vi "UpdateZones.vi"(0 "object in":refnum<class "Team.lvclass">, 2 "Robots":refnum<class "Robot.lvclass">[](array[class]), 5 "error in (no error)":errorcluster) -> (14 "object out":refnum<class "Team.lvclass">, 19 "error out":errorcluster)   [LabVIEW 2023, in "Team.lvclass"]
uses:
  Team.lvclass
  Robot_class/Robot.lvclass
  Team.lvclass/Team.ctl
  Zone_class/Zone.lvclass
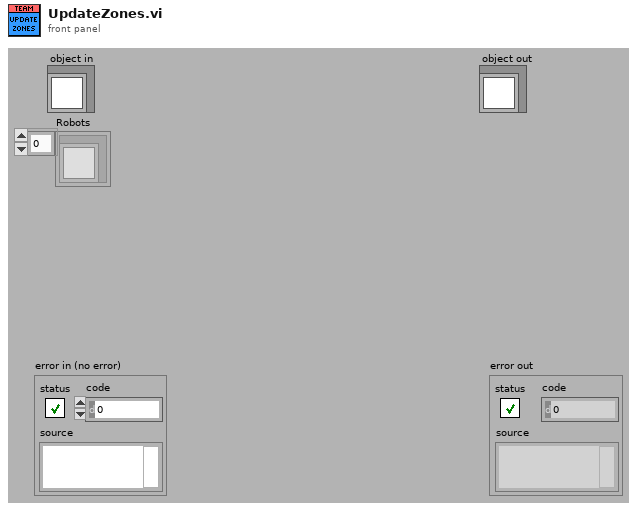
[diagram p1: front panel]
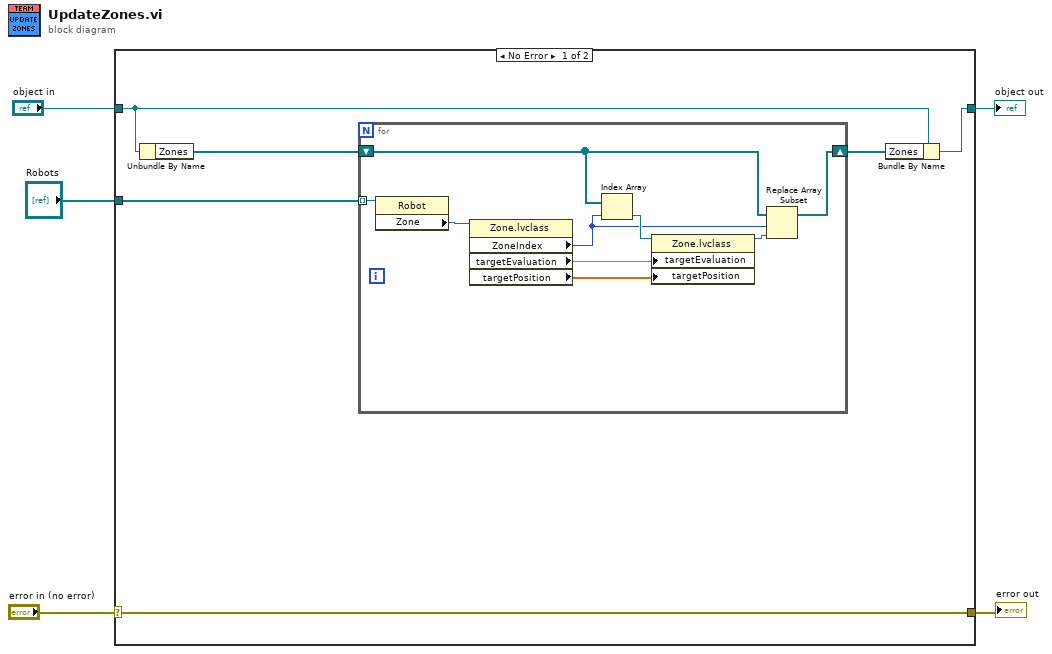
[diagram p0: block diagram]
diagram:
  n1 = case shown="No Error" "error in (no error)" {
    selector: "error in (no error)" -> [w11 w22]
    tunnel: [w11 w22] -> w4
    tunnel: [w6 w21] -> w2
    tunnel: "object in" -> [w7 w21]
    tunnel: "Robots" -> [w10 _]
    frame No Error {
      n2 = Unbundle By Name(w7) -> ("Zones"=w9:refnum<class "Zone.lvclass">[])
      n3 = for {
        tunnel: w10 -> [w20] mode=indexing
        shift-right: [w13] -> w8
        shift-left: w9 -> [w14]
        n4 = property class="Robot"(reference=w20) -> ("Zone"=w18:refnum<class "Zone.lvclass">)  [unwired: 1 in, 2 out]
        n5 = property class="Zone.lvclass"(reference=w18) -> ("ZoneIndex"=w12:i32, "targetEvaluation"=w17:dbl, "targetPosition"=w16:dbl[])  [unwired: 1 in, 2 out]
        n6 = Index Array(array=w14, index=w12) -> (element=w19:refnum<class "Zone.lvclass">)
        n7 = property class="Zone.lvclass"(reference=w19, "targetEvaluation"=w17, "targetPosition"=w16) -> (reference out=w15:refnum<class "Zone.lvclass">)  [unwired: 1 in, 1 out]
        n8 = Replace Array Subset(array=w14, new element=w15, index=w12) -> (w13:refnum<class "Zone.lvclass">[])
      }
      n9 = Bundle By Name(cluster=w7, "Zones"=w8) -> (w6:refnum<class "Team.lvclass">)
    }
    frame Error {
    }
  }
  "error out" <- w4
  "object out" <- w2
